vi "Osc Trigger.vi"(0 "RedPitaya connection in":refnum<k5>, 1 "Trigger Sweep":string(combo), 2 "Trigger Source":string(combo), 3 "Trigger Slope":string(combo), 4 "Trigger Level":dbl=21.0 min=-20.0 max=21.0, 5 "error in":errorcluster, 12 "timeout ms (2000)":i32=2000) -> (14 "RedPitaya connection out":refnum<k5>, 19 "error out":errorcluster)   [LabVIEW 2010, in "RedPitaya.lvlib"]
doc: "Configures oscilloscope trigger parameters"
uses:
  RedPitaya.lvlib
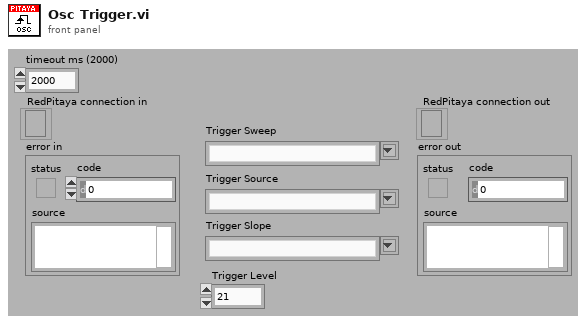
[diagram p1: front panel]
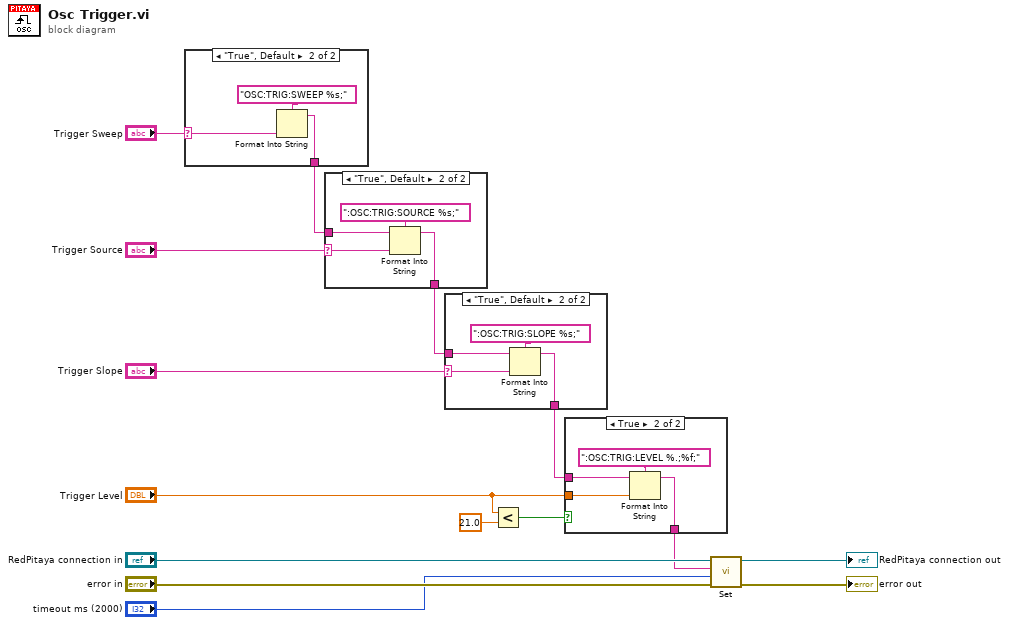
[diagram p0: block diagram]
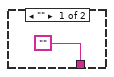
[diagram p5: hidden frame]
diagram:
  n1 = case shown="\"True\", Default" "Trigger Sweep" {
    selector: "Trigger Sweep" -> [_ w17]
    tunnel: ["" w18] -> w11
    frame "" {
    }
    frame "True", Default {
      n2 = Format Into String(format string="OSC:TRIG:SWEEP %s;", w17) -> (resulting string=w18:string)  [unwired: 2 in, 1 out]
    }
  }
  n3 = case shown="\"True\", Default" "Trigger Source" {
    selector: "Trigger Source" -> [_ w21]
    tunnel: w11 -> [w20 w24]
    tunnel: [w20 w22] -> w8
    frame "" {
    }
    frame "True", Default {
      n4 = Format Into String(format string=":OSC:TRIG:SOURCE %s;", initial string=w24, w21) -> (resulting string=w22:string)  [unwired: 1 in, 1 out]
    }
  }
  n5 = case shown="\"True\", Default" "Trigger Slope" {
    selector: "Trigger Slope" -> [_ w26]
    tunnel: w8 -> [w25 w29]
    tunnel: [w25 w27] -> w6
    frame "" {
    }
    frame "True", Default {
      n6 = Format Into String(format string=":OSC:TRIG:SLOPE %s;", initial string=w29, w26) -> (resulting string=w27:string)  [unwired: 1 in, 1 out]
    }
  }
  n7 = Less?(x="Trigger Level", y=21.0) -> (x < y?=w5:bool)
  n8 = case shown="True" w5 {
    tunnel: w6 -> [w30 w34]
    tunnel: [w30 w32] -> w2
    tunnel: "Trigger Level" -> [_ w31]
    frame False {
    }
    frame True, Default {
      n9 = Format Into String(format string=":OSC:TRIG:LEVEL %.;%f;", initial string=w34, w31) -> (resulting string=w32:string)  [unwired: 1 in, 1 out]
    }
  }
  n10 = call "Set.vi"("error in"="error in", "timeout ms (2000)"="timeout ms (2000)", "SCPI Message"=w2, "RedPitaya connection in"="RedPitaya connection in") -> ("error out"=→"error out":errorcluster, "RedPitaya connection out"=→"RedPitaya connection out":refnum<k5>)  [unwired: 5 in, 1 out]
